vi "BNC555.Revision Query.vi"(0 "i ref in":refnum<vi>, 5 "error IO":errorcluster) -> (14 "i ref out":refnum<vi>, 19 "error out":errorcluster)   [LabVIEW 2014, in "BNC555.lvlib"]
doc: "This VI queries hard- and software for the current revision and displays the information at the GUI."
uses:
  BNC555.lvlib
  CS_PHELIX/PH_Basics/PH_Common/PH_Common.lvlib
  instr.lib/BNC555/BNC555 - Driver np.lvlib
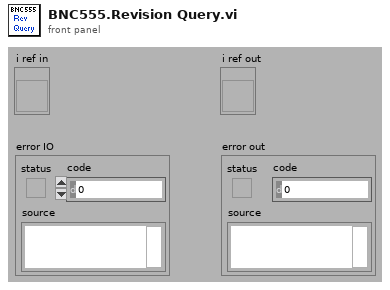
[diagram p1: front panel]
types:
  T1 = typedef "BNC555.lvlib/BNC555.i attribute.ctl" = cluster{"Information":cluster{"VISA resource name":refnum<visa-resource-name>, "Baud Rate (1:9600)":u16}, "Channel Array":T2[], "System":T3, "GUI Refs":cluster{"Delete":refnum<vi>, "Information":refnum<vi>, "System":refnum<vi>, "Channel Array":refnum<vi>, "Device Error":refnum<vi>, "Instr Driver Revision":refnum<vi>, "Instr Firmware Revision":refnum<vi>, "Instr Option":refnum<vi>, "Self-Test Response":refnum<vi>}, "Service IDs Channelinfo":i32[], "Service ID T0 Mode":i32}
  T2 = typedef "BNC555 - Driver np.lvlib/BNC555 All Chan Parameters.ctl" = cluster{"Chan #":i32, "Chan State":bool, "Chan Delay":dbl, "Chan Width":dbl, "Chan Mode":enum16{"Normal", "Single", "Burst", "Divide by N"}, "Chan Burst #":u32, "Chan Divide #":u32, "Chan Pol Out":enum16{"Normal", "Complement", "Inverted"}, "Chan Level Out":enum16{"TTL", "Adjustable", "35 Volt"}, "Chan Lev Adjust":dbl, "Chan Gate Pol":enum16{"Normal", "Complement", "Inverted"}, "Chan Gate State":bool}
  T3 = typedef "BNC555 - Driver np.lvlib/BNC555 All Sys Parameters.ctl" = cluster{"Sys Period":dbl, "Sys Oscillator":bool, "Sys Mode":enum16{"Normal", "Single", "Burst", "Duty Cycle"}, "Sys Burst #":u32, "Sys DC On":u32, "Sys DC Off":u32, "Sys Trig Mode":enum16{"Disabled", "Triggered", "Gated"}, "Sys Trig Lev":dbl, "Sys Gate State":bool, "Sys Trig Edge":bool, "Sys State":bool}
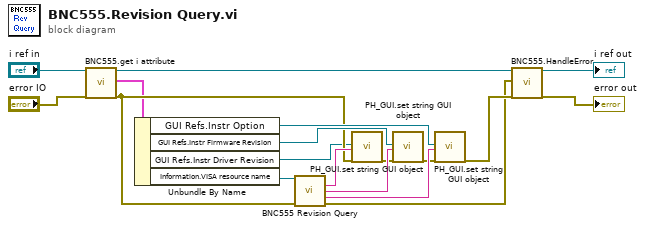
[diagram p0: block diagram]
diagram:
  n1 = call "BNC555.get i attribute.vi"("i ref in"="i ref in", "error in (no error)"="error IO") -> ("i ref out"=w6:refnum<vi>, "i attribute"=w5:T1, "error out"=w8:errorcluster)  [unwired: 15 in]
  n2 = Unbundle By Name(w5) -> ("GUI Refs.Instr Option"=w18:refnum<vi>, "GUI Refs.Instr Firmware Revision"=w17:refnum<vi>, "GUI Refs.Instr Driver Revision"=w7:refnum<vi>, "Information.VISA resource name"=w10:refnum<visa-resource-name>)
  n3 = call "BNC555 Revision Query.vi"("VISA resource"=w10, "error in (no error)"=w8) -> ("Instr Driver Revision"=w11:string, "Instr Firmware Revision"=w15:string, "Instr Option"=w16:string, "error out"=w9:errorcluster)  [unwired: 9 in, 1 out]
  n4 = call "PH_GUI.set string GUI object.vi"("GUI object Ref"=w7, "Text"=w11, "error in"=w8) -> ("error out"=w13:errorcluster)  [unwired: 16 in]
  n5 = call "PH_GUI.set string GUI object.vi"("GUI object Ref"=w17, "Text"=w15, "error in"=w13) -> ("error out"=w12:errorcluster)  [unwired: 16 in]
  n6 = call "PH_GUI.set string GUI object.vi"("GUI object Ref"=w18, "Text"=w16, "error in"=w12) -> ("error out"=w14:errorcluster)  [unwired: 16 in]
  n7 = call "BNC555.HandleError.vi"("i ref in"=w6, "Device error"=w9, "error in (no error)"=w14) -> ("i ref out"=→"i ref out":refnum<vi>, "error out"=→"error out":errorcluster)  [unwired: 15 in]
